vi "Write Next channel idx.vi"(8 "error in (no error)":errorcluster, 10 "Next channel idx":i32, 11 "Channel Scanner Driver in":refnum<class "Channel Scanner Driver.lvclass">) -> (0 "error out":errorcluster, 3 "Channel Scanner Driver out":refnum<class "Channel Scanner Driver.lvclass">)   [LabVIEW 2019, in "Channel Scanner Driver.lvclass"]
uses:
  Channel Scanner Driver.lvclass
  Channel Scanner Driver.lvclass/Channel Scanner Driver.ctl
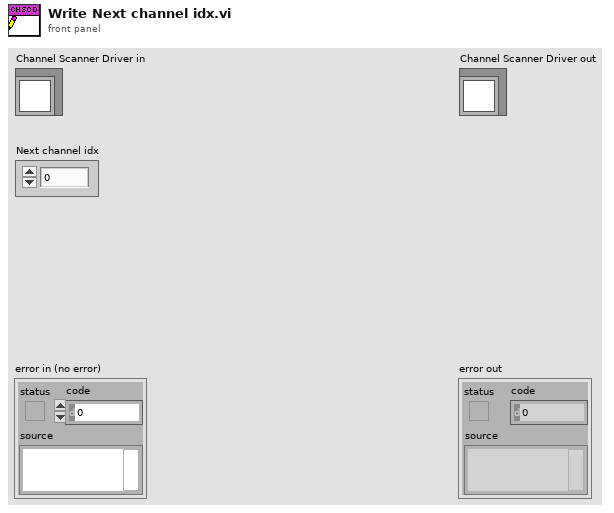
[diagram p1: front panel]
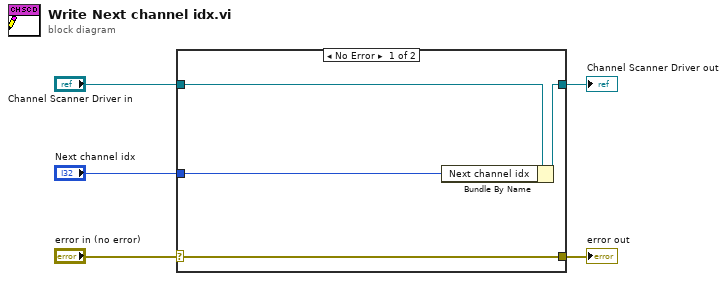
[diagram p0: block diagram]
diagram:
  n1 = case shown="No Error" "error in (no error)" {
    selector: "error in (no error)" -> [w9 w10]
    tunnel: [w9 w10] -> w4
    tunnel: [w7 w11] -> w2
    tunnel: "Channel Scanner Driver in" -> [w8 w11]
    tunnel: "Next channel idx" -> [w6 _]
    frame No Error {
      n2 = Bundle By Name(cluster=w8, "Next channel idx"=w6) -> (w7:refnum<class "Channel Scanner Driver.lvclass">)
    }
    frame Error {
    }
  }
  "error out" <- w4
  "Channel Scanner Driver out" <- w2
